vi "Get Type.vi"(8 "error in (no error)":errorcluster, 11 "Single Cell Battery in":refnum<class "Single Cell Battery.lvclass">) -> (0 "error out":errorcluster, 2 "Item Type":T1, 3 "Single Cell Battery out":refnum<class "Single Cell Battery.lvclass">)   [LabVIEW 2020, in "Single Cell Battery.lvclass"]
uses:
  Single Cell Battery.lvclass
  Item/Item Type.ctl
  Item/Item.lvclass
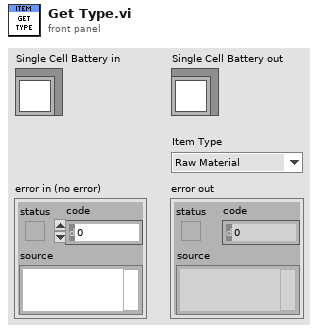
[diagram p1: front panel]
types:
  T1 = typedef "Item.lvclass/Item Type.ctl" = enum16{"Raw Material", "Component", "Module", "Product"}
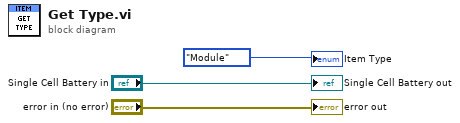
[diagram p0: block diagram]
diagram:
  "error out" <- "error in (no error)"
  "Single Cell Battery out" <- "Single Cell Battery in"
  "Item Type" <- Item_Type."Module" ("Item Type")
